vi "Validate Connection.vi"(8 "error in (no error)":errorcluster, 11 "VISA Refnum in":refnum<visa-resource-name>) -> (0 "error out":errorcluster, 3 "VISA Refnum out":refnum<visa-resource-name>)   [LabVIEW 2019, in "KH7008.lvlib"]
uses:
  KH7008.lvlib
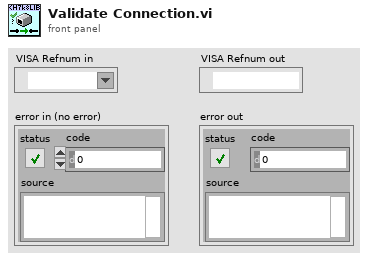
[diagram p1: front panel]
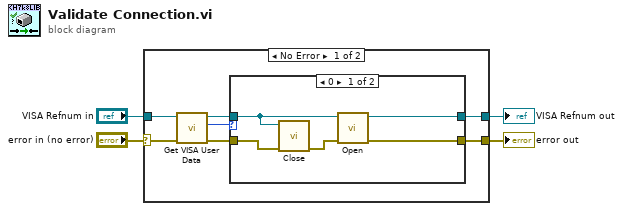
[diagram p0: block diagram]
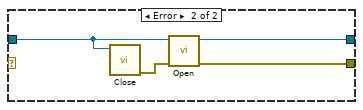
[diagram p3: hidden frame]
diagram:
  n1 = case shown="No Error" "error in (no error)" {
    selector: "error in (no error)" -> [w5 _]
    tunnel: [w11 w20] -> w4
    tunnel: "VISA Refnum in" -> [w9 w21]
    tunnel: [w10 w19] -> w2
    frame No Error {
      n2 = call "Get VISA User Data.vi"("error in (no error)"=w5, "VISA Refnum in"=w9) -> ("error out"=w6:errorcluster, "User Data"=w7:i32, "VISA Refnum out"=w8:refnum<visa-resource-name>)  [unwired: 7 in]
      n3 = case shown="0" w7 {
        tunnel: [w13 w18] -> w11
        tunnel: w6 -> [w15 w17]
        tunnel: w8 -> [w14 w18]
        tunnel: [w12 w17] -> w10
        frame 0 {
          n4 = call "Close.vi"("error in (no error)"=w15, "VISA resource name"=w14) -> ("error out"=w16:errorcluster)  [unwired: 9 in]
          n5 = call "Open.vi"("error in (no error)"=w16, "VISA resource name"=w14) -> ("error out"=w12:errorcluster, "VISA resource"=w13:refnum<visa-resource-name>)  [unwired: 8 in]
        }
        frame Default {
        }
      }
    }
    frame Error {
      n6 = call "Close.vi"("VISA resource name"=w21) -> ("error out"=w22:errorcluster)  [unwired: 10 in]
      n7 = call "Open.vi"("error in (no error)"=w22, "VISA resource name"=w21) -> ("error out"=w19:errorcluster, "VISA resource"=w20:refnum<visa-resource-name>)  [unwired: 8 in]
    }
  }
  "VISA Refnum out" <- w4
  "error out" <- w2
